vi "ASI Get Camera Property.vi"(10 "iCameraIndex":i32, 11 "pASICameraInfo":T1 {"IsColorCam" items=["ASI_FALSE", "ASI_TRUE"]; "BayerPattern" items=["ASI_BAYER_RG", "ASI_BAYER_BG", "ASI_BAYER_GR", "ASI_BAYER_GB"]; "MechanicalShutter" items=["ASI_FALSE", "ASI_TRUE"]; "ST4Port" items=["ASI_FALSE", "ASI_TRUE"]; "IsCoolerCam" items=["ASI_FALSE", "ASI_TRUE"]; "IsUSB3Host" items=["ASI_FALSE", "ASI_TRUE"]; "IsUSB3Camera" items=["ASI_FALSE", "ASI_TRUE"]}) -> (0 "supportedBin":i8[](array[numeric]), 1 "supportedImgType":i8[](array[numeric]), 2 "function return":i32, 3 "pASICameraInfo out":T1 {"IsColorCam" items=["ASI_FALSE", "ASI_TRUE"]; "BayerPattern" items=["ASI_BAYER_RG", "ASI_BAYER_BG", "ASI_BAYER_GR", "ASI_BAYER_GB"]; "MechanicalShutter" items=["ASI_FALSE", "ASI_TRUE"]; "ST4Port" items=["ASI_FALSE", "ASI_TRUE"]; "IsCoolerCam" items=["ASI_FALSE", "ASI_TRUE"]; "IsUSB3Host" items=["ASI_FALSE", "ASI_TRUE"]; "IsUSB3Camera" items=["ASI_FALSE", "ASI_TRUE"]}, 8 "cameraName":string)   [LabVIEW 2023, in "ASICamera2_no_err.lvlib"]
doc: "ASICAMERA_API ASI_ERROR_CODE ASIGetCameraProperty(ASI_CAMERA_INFO *pASICameraInfo, int iCameraIndex);"
uses:
  ASICamera2_no_err.lvlib
  LabviewDAQ-master/ConcreteClasses/ConcreteInstrumentClasses/CameraClasses/ZWO_ASI_LV/Labview_ASI_demo_64bit_221128/user.lib/ASICamera2_no_err/ASICamera2.dll
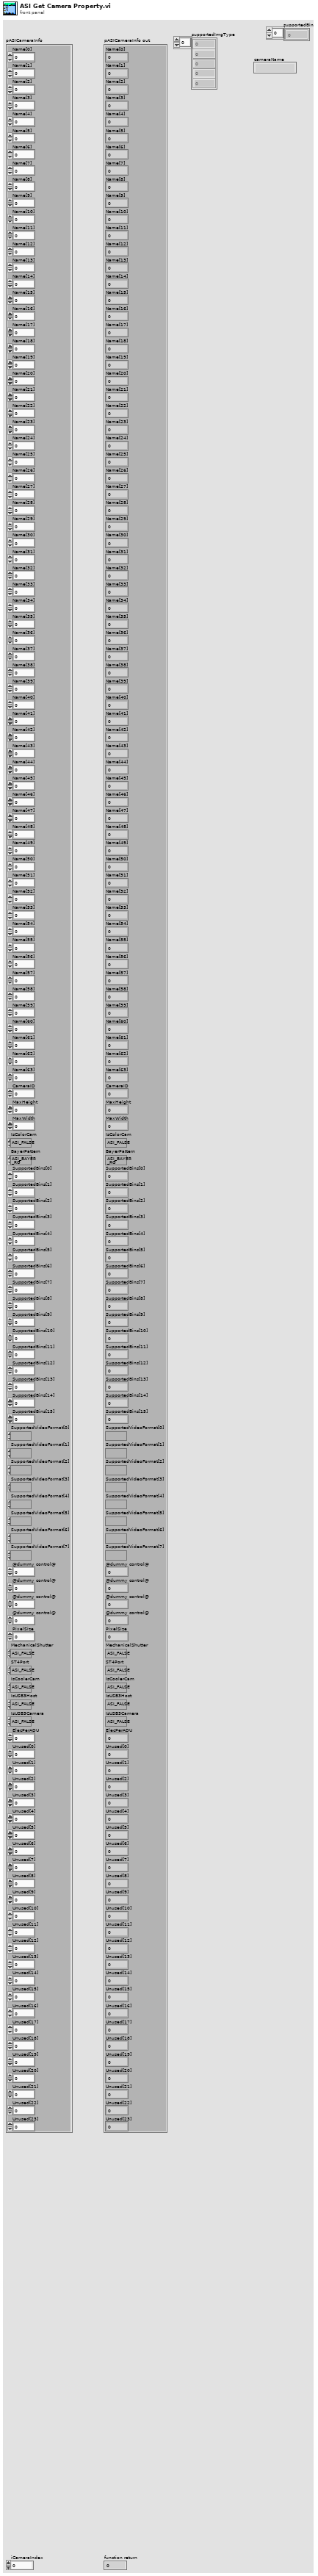
[diagram p1: front panel]
types:
  T1 = cluster{"Name[0]":i8, "Name[1]":i8, "Name[2]":i8, "Name[3]":i8, "Name[4]":i8, "Name[5]":i8, "Name[6]":i8, "Name[7]":i8, "Name[8]":i8, "Name[9]":i8, "Name[10]":i8, "Name[11]":i8, "Name[12]":i8, "Name[13]":i8, "Name[14]":i8, "Name[15]":i8, "Name[16]":i8, "Name[17]":i8, "Name[18]":i8, "Name[19]":i8, "Name[20]":i8, "Name[21]":i8, "Name[22]":i8, "Name[23]":i8, "Name[24]":i8, "Name[25]":i8, "Name[26]":i8, "Name[27]":i8, "Name[28]":i8, "Name[29]":i8, "Name[30]":i8, "Name[31]":i8, "Name[32]":i8, "Name[33]":i8, "Name[34]":i8, "Name[35]":i8, "Name[36]":i8, "Name[37]":i8, "Name[38]":i8, "Name[39]":i8, "Name[40]":i8, "Name[41]":i8, "Name[42]":i8, "Name[43]":i8, "Name[44]":i8, "Name[45]":i8, "Name[46]":i8, "Name[47]":i8, "Name[48]":i8, "Name[49]":i8, "Name[50]":i8, "Name[51]":i8, "Name[52]":i8, "Name[53]":i8, "Name[54]":i8, "Name[55]":i8, "Name[56]":i8, "Name[57]":i8, "Name[58]":i8, "Name[59]":i8, "Name[60]":i8, "Name[61]":i8, "Name[62]":i8, "Name[63]":i8, "CameraID":i32, "MaxHeight":i32, "MaxWidth":i32, "IsColorCam":u32, "BayerPattern":u32, "SupportedBins[0]":i32, "SupportedBins[1]":i32, "SupportedBins[2]":i32, "SupportedBins[3]":i32, "SupportedBins[4]":i32, "SupportedBins[5]":i32, "SupportedBins[6]":i32, "SupportedBins[7]":i32, "SupportedBins[8]":i32, "SupportedBins[9]":i32, "SupportedBins[10]":i32, "SupportedBins[11]":i32, "SupportedBins[12]":i32, "SupportedBins[13]":i32, "SupportedBins[14]":i32, "SupportedBins[15]":i32, "SupportedVideoFormat[0]":u32, "SupportedVideoFormat[1]":u32, "SupportedVideoFormat[2]":u32, "SupportedVideoFormat[3]":u32, "SupportedVideoFormat[4]":u32, "SupportedVideoFormat[5]":u32, "SupportedVideoFormat[6]":u32, "SupportedVideoFormat[7]":u32, "@dummy control@":i8, "@dummy control@":i8, "@dummy control@":i8, "@dummy control@":i8, "PixelSize":dbl, "MechanicalShutter":u32, "ST4Port":u32, "IsCoolerCam":u32, "IsUSB3Host":u32, "IsUSB3Camera":u32, "ElecPerADU":sgl, "Unused[0]":i8, "Unused[1]":i8, "Unused[2]":i8, "Unused[3]":i8, "Unused[4]":i8, "Unused[5]":i8, "Unused[6]":i8, "Unused[7]":i8, "Unused[8]":i8, "Unused[9]":i8, "Unused[10]":i8, "Unused[11]":i8, "Unused[12]":i8, "Unused[13]":i8, "Unused[14]":i8, "Unused[15]":i8, "Unused[16]":i8, "Unused[17]":i8, "Unused[18]":i8, "Unused[19]":i8, "Unused[20]":i8, "Unused[21]":i8, "Unused[22]":i8, "Unused[23]":i8}
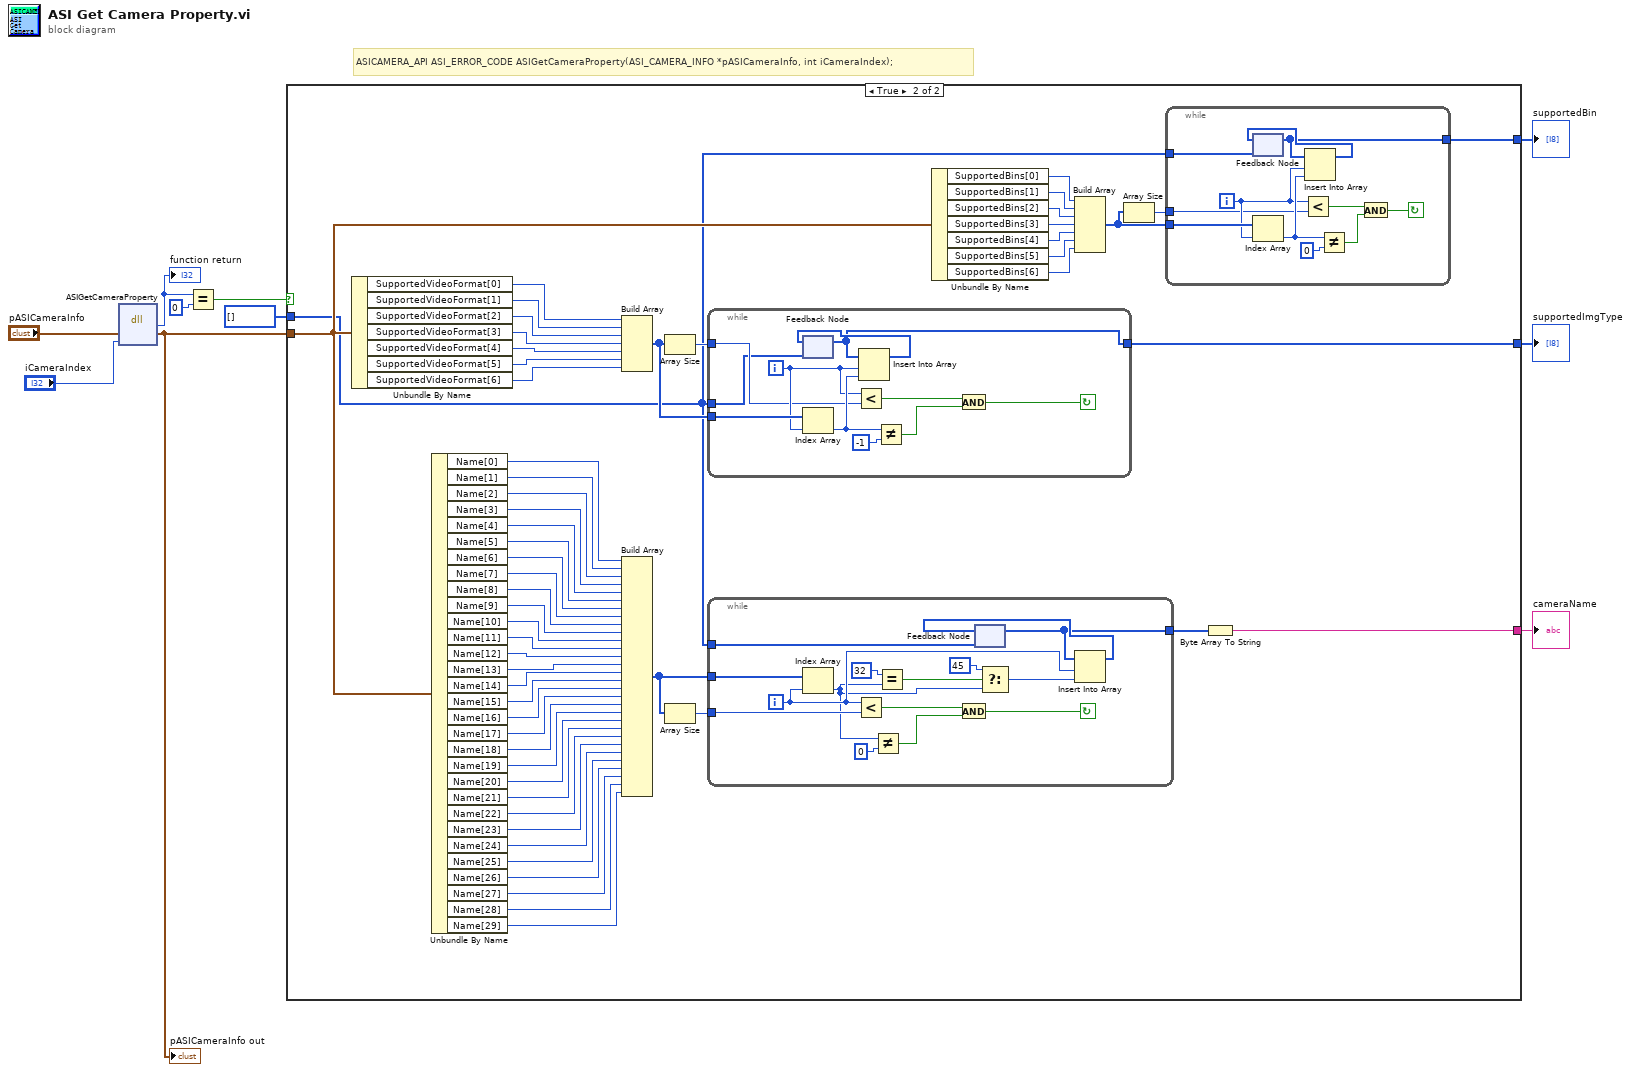
[diagram p0: block diagram]
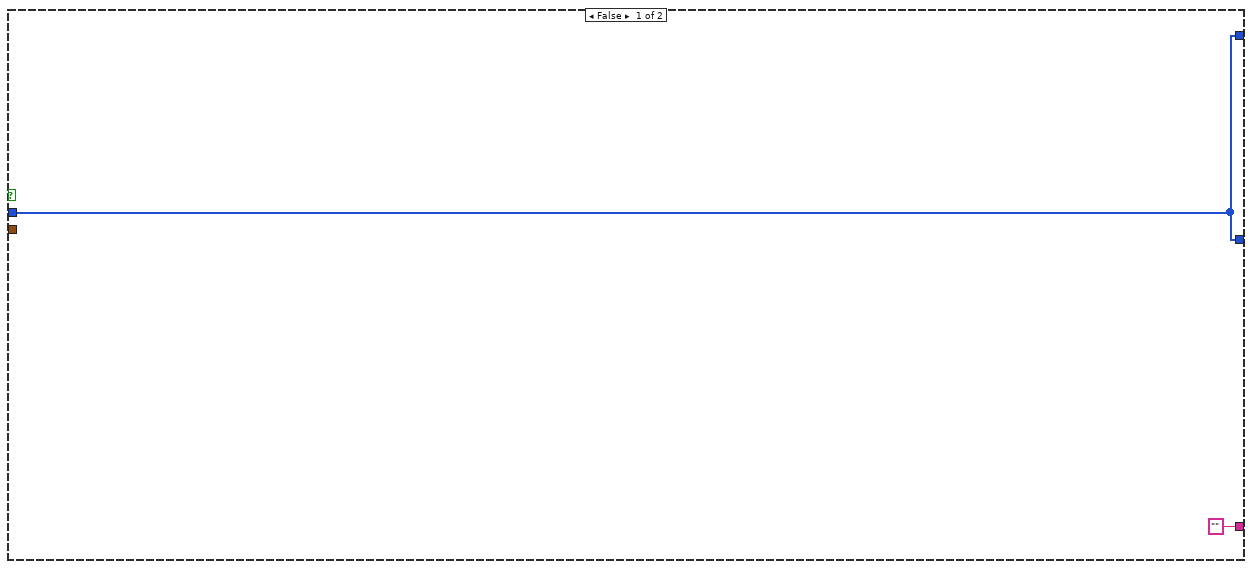
[diagram p2: hidden frame]
diagram:
  # "ASICAMERA_API ASI_ERROR_CODE ASIGetCameraProperty(ASI_CAMERA_INFO *pASICameraInfo, int iCameraIndex);"
  n1 = dll-call lib="W:/Quant_Opt_Group/Group/Alex/LabviewDAQ-master/ConcreteClasses/ConcreteInstrumentClasses/CameraClasses/ZWO_ASI_LV/Labview_ASI_demo_64bit_221128/user.lib/ASICamera2_no_err/ASICamera2.*" fn="ASIGetCameraProperty"("pASICameraInfo"="pASICameraInfo", "iCameraIndex"="iCameraIndex") -> (w6:i32, "pASICameraInfo"=w8:T1)  [unwired: 4 in, 2 out]
  "function return" <- w6
  "pASICameraInfo out" <- w8
  n2 = Equal?(x=w6, y=0) -> (x = y?=w4:bool)
  n3 = case shown="True" w4 {
    tunnel: w8 -> [_ w48]
    tunnel: [w12 w61] -> w7
    tunnel: i8[] [] -> [w12 w16]
    tunnel: [w12 w49] -> w2
    tunnel: ["" ("string") w17] -> w1
    frame False {
    }
    frame True {
      n4 = Unbundle By Name(w48) -> ("SupportedVideoFormat[0]"=w68:u32, "SupportedVideoFormat[1]"=w67:u32, "SupportedVideoFormat[2]"=w66:u32, "SupportedVideoFormat[3]"=w65:u32, "SupportedVideoFormat[4]"=w64:u32, "SupportedVideoFormat[5]"=w63:u32, "SupportedVideoFormat[6]"=w62:u32)
      n5 = Unbundle By Name(w48) -> ("Name[0]"=w47:i8, "Name[1]"=w46:i8, "Name[2]"=w45:i8, "Name[3]"=w44:i8, "Name[4]"=w43:i8, "Name[5]"=w42:i8, "Name[6]"=w41:i8, "Name[7]"=w40:i8, "Name[8]"=w39:i8, "Name[9]"=w38:i8, "Name[10]"=w37:i8, "Name[11]"=w36:i8, "Name[12]"=w35:i8, "Name[13]"=w34:i8, "Name[14]"=w33:i8, "Name[15]"=w32:i8, "Name[16]"=w31:i8, "Name[17]"=w30:i8, "Name[18]"=w29:i8, "Name[19]"=w28:i8, "Name[20]"=w27:i8, "Name[21]"=w26:i8, "Name[22]"=w25:i8, "Name[23]"=w24:i8, "Name[24]"=w23:i8, "Name[25]"=w22:i8, "Name[26]"=w21:i8, "Name[27]"=w20:i8, "Name[28]"=w19:i8, "Name[29]"=w18:i8)
      n6 = Build Array(w68, w67, w66, w65, w64, w63, w62) -> (w60:u32[])
      n7 = Build Array(w47, w46, w45, w44, w43, w42, w41, w40, w39, w38, w37, w36, w35, w34, w33, w32, w31, w30, w29, w28, w27, w26, w25, w24, w23, w22, w21, w20, w19, w18) -> (w14:i8[])
      n8 = Array Size(array=w60) -> (size(s)=w59:i32)
      n9 = Array Size(array=w14) -> (size(s)=w15:i32)
      n10 = while {
        tunnel: [w101] -> w61
        tunnel: w60 -> [w103]
        tunnel: w59 -> [w99]
        tunnel: w16 -> [w95]
        i -> [w100]
        stop <- w96 continue-if-true
        n11 = feedback #1(w95) -> (w101:i8[])
        n12 = Index Array(array=w103, index=w100) -> (element=w105:u32)
        n13 = Less?(x=w100, y=w99) -> (x < y?=w97:bool)
        n14 = Insert Into Array(array=w101, index=w100, new element=w105) -> (w102:i8[])
        n15 = feedback-in #1(w102) -> ()
        n16 = Not Equal?(x=w105, y=i8 -1) -> (x != y?=w98:bool)
        n17 = And(x=w97, y=w98) -> (x .and. y?=w96:bool)
      }
      n18 = while {
        tunnel: [w81] -> w13
        tunnel: w14 -> [w76]
        tunnel: w15 -> [w75]
        tunnel: w16 -> [w74]
        i -> [w80]
        stop <- w77 continue-if-true
        n19 = Index Array(array=w76, index=w80) -> (element=w69:i8)
        n20 = Less?(x=w80, y=w75) -> (x < y?=w78:bool)
        n21 = Not Equal?(x=w69, y=i8 0) -> (x != y?=w79:bool)
        n22 = Equal?(x=i8 32, y=w69) -> (x = y?=w72:bool)
        n23 = And(x=w78, y=w79) -> (x .and. y?=w77:bool)
        n24 = feedback #2(w74) -> (w81:i8[])
        n25 = Select(t=i8 45, s=w72, f=w69) -> (s? t:f=w70:i8)
        n26 = Insert Into Array(array=w81, index=w80, new element=w70) -> (w82:i8[])
        n27 = feedback-in #2(w82) -> ()
      }
      n28 = Unbundle By Name(w48) -> ("SupportedBins[0]"=w58:i32, "SupportedBins[1]"=w57:i32, "SupportedBins[2]"=w56:i32, "SupportedBins[3]"=w55:i32, "SupportedBins[4]"=w54:i32, "SupportedBins[5]"=w53:i32, "SupportedBins[6]"=w52:i32)
      n29 = Build Array(w58, w57, w56, w55, w54, w53, w52) -> (w51:i32[])
      n30 = Array Size(array=w51) -> (size(s)=w50:i32)
      n31 = while {
        tunnel: [w90] -> w49
        tunnel: w51 -> [w92]
        tunnel: w50 -> [w88]
        tunnel: w16 -> [w84]
        i -> [w89]
        stop <- w85 continue-if-true
        n32 = feedback #3(w84) -> (w90:i8[])
        n33 = Index Array(array=w92, index=w89) -> (element=w94:i32)
        n34 = Less?(x=w89, y=w88) -> (x < y?=w86:bool)
        n35 = Insert Into Array(array=w90, index=w89, new element=w94) -> (w91:i8[])
        n36 = feedback-in #3(w91) -> ()
        n37 = Not Equal?(x=w94, y=i8 0) -> (x != y?=w87:bool)
        n38 = And(x=w86, y=w87) -> (x .and. y?=w85:bool)
      }
      n39 = Byte Array To String(unsigned byte array=w13) -> (string=w17:string)
    }
  }
  "supportedImgType" <- w7
  "supportedBin" <- w2
  "cameraName" <- w1
